vi "Fit Decay with Offset v2.vi"(0 "Y Array":dbl[](array[numeric]), 1 "X Array":dbl[](array[numeric]), 2 "Weights":dbl[](array[numeric]), 3 "Initial Parameters":dbl[](array[numeric]), 4 "Decay Fit Options":T2={"Show Fit Residuals"=TRUE, "Fit Model"=enum."1-Exponential", "Residual Type"=enum."Standard", "Max Decay Percentile"=0.0, "Min Decay Percentile"=0.0, "Show Full Decay"=TRUE, "Weights"=enum."Unweighted", "Fitting Method"=enum."Least Square", "Compute Parameter Uncertainties"=TRUE, "Periodic Boundaries"=TRUE, "Model Calculation"=enum."Simulation", "Period"=1.2500000000000001e-08, "Termination Criteria"={"Max Iterations"=0, "Max Function Calls"=0, "Max Time"=1000.0, "Function Tolerance"=1e-06, "Parameter Tolerance"=1e-06, "Gradient Tolerance"=0.0, "Min Lambda"=1e-06, "Max Lambda"=1e-06, "Initial Tick Count"=0}, "Offset Resolution"=1.2500000000000001e-08, "Use Local IRF"=TRUE, "Fitting Algorithm"=enum."Levenberg-Marquardt", "Show Confidence Interval "=TRUE, "Confidence Level"=95.0} {"Confidence Level" min=0.0 max=100.0; "Offset Resolution" min=0.0; "Period" min=0.0; "Min Decay Percentile" min=0.0 max=1.0; "Max Decay Percentile" min=0.0 max=100.0}, 5 "error in (no error)":errorcluster, 6 "f(x,a)":refnum<vi>, 7 "parameter bounds":T15, 8 "Data":variant, 9 "Decay Normalization Factor":dbl, 10 "Model Name":string, 11 "IRF Normalization Factor":dbl, 12 "Optimal Offset Selection Criterion":T1) -> (14 "Fit Output":T10={"best nonlinear fit"=[], "best fit parameters"=[], "R^2"=0.0, "RMSE"=0.0, "error out"={"status"=FALSE, "code"=0, "source"=""}, "Fitting Method"=enum."Least Square", "number of function calls"=0, "number of iterations"=0, "covariance"=[], "Chi 2"=0.0, "DOF"=0, "Fit Convergence Criterion"=enum."Continue", "Fitting Algorithm"=enum."Levenberg-Marquardt", "Weighted Fit"=enum."Unweighted", "Gradient"=0.0, "|Delta Chi 2|"=0.0, "|Delta Chi 2|/Chi 2"=0.0, "Max |Delta a| /|a|"=0.0, "Lambda"=-1.0, "RSS"=0.0, "AIC"=0.0, "BIC"=0.0, "Max number of function calls"=0, "Max number of iterations"=0, "IRF"={"X Array"=[], "Y Array"=[]}, "IRF Normalization Factor"=0.0, "Decay Normalization Factor"=0.0, "Number of offset fits"=0, "Weighted Chi2"=-1.0, "Unweighted Chi2"=-1.0}, 15 "Fit Aborted?":bool, 17 "Fit Results (Stats)":T9[](array[typedef]), 18 "C_00":dbl, 19 "error out":errorcluster)   [LabVIEW 2021, in "Fits.lvlib"]
uses:
  Fits.lvlib
  Non-linear Fit Output v4.ctl
  Nonlinear Fit Method.ctl
  <vilib>/Analysis/Matrix/Datatypes/RealMatrix.ctl
  Convergence Criteria.ctl
  Non-linear Fitting Algorithm.ctl
  Fit Weights Type v2.ctl
  Graphs/XY Graph/XY Graph Plot Data.ctl
  Fit Results (statistics).ctl
  Non-linear Fitting Method v2.ctl
  Decay Fit Options v4.ctl
  Decay Convolution/Decay Model.ctl
  Residual Type.ctl
  Fit Calculation Method.ctl
  Optimal Offset Selection Criterion.ctl
  Decay Fit Steps.ctl
  <vilib>/Analysis/Matrix/NI_Matrix.lvlib
  Graphs/XY Graph/XY Graph Add-Ons.lvlib
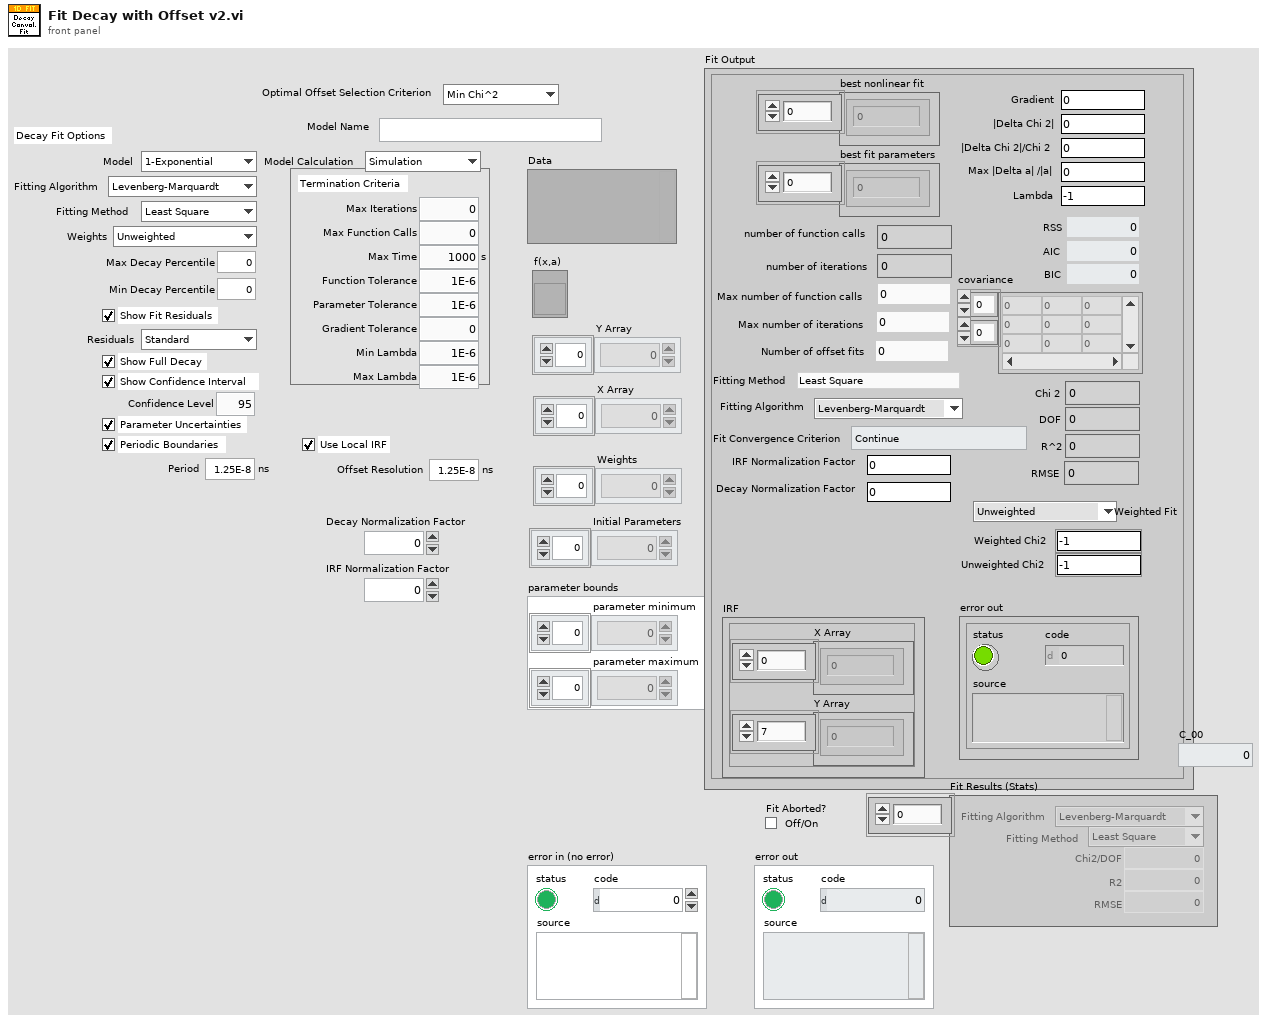
[diagram p1: front panel]
types:
  T1 = typedef "Fits.lvlib/Optimal Offset Selection Criterion.ctl" = enum16{"Min Chi^2", "Max R^2"}
  T2 = typedef "Fits.lvlib/Decay Fit Options v4.ctl" = cluster{"Show Fit Residuals":bool, "Fit Model":T3, "Residual Type":T4, "Max Decay Percentile":dbl, "Min Decay Percentile":dbl, "Show Full Decay":bool, "Weights":T5, "Fitting Method":T6, "Compute Parameter Uncertainties":bool, "Periodic Boundaries":bool, "Model Calculation":T7, "Period":dbl[unit], "Termination Criteria":cluster{"Max Iterations":i32, "Max Function Calls":i32, "Max Time":dbl[unit], "Function Tolerance":dbl, "Parameter Tolerance":dbl, "Gradient Tolerance":dbl, "Min Lambda":dbl, "Max Lambda":dbl, "Initial Tick Count":u32}, "Offset Resolution":dbl[unit], "Use Local IRF":bool, "Fitting Algorithm":T8, "Show Confidence Interval ":bool, "Confidence Level":dbl}
  T3 = typedef "Fits.lvlib/Decay Model.ctl" = enum16{"1-Exponential", "2-Exponentials"}
  T4 = typedef "Fits.lvlib/Residual Type.ctl" = enum16{"Standard", "Normalized", "Reduced"}
  T5 = typedef "Fits.lvlib/Fit Weights Type v2.ctl" = enum16{"Unweighted", "1/Variance (Neyman)", "1/Variance (Pearson)", "Best of All"}
  T6 = typedef "Fits.lvlib/Non-linear Fitting Method v2.ctl" = enum16{"Least Square", "Least Absolute Residual", "Bisquare", "MLE", "-", "Best of All"}
  T7 = typedef "Fits.lvlib/Fit Calculation Method.ctl" = enum16{"Simulation", "Convolution", "Integration"}
  T8 = typedef "Fits.lvlib/Non-linear Fitting Algorithm.ctl" = enum16{"Levenberg-Marquardt", "Trust-Region Dogleg"}
  T9 = typedef "Fits.lvlib/Fit Results (statistics).ctl" = cluster{"Chi2/DOF":dbl, "R2":dbl, "RMSE":dbl, "Fitting Method":T6, "Fitting Algorithm":T8}
  T10 = typedef "Fits.lvlib/Non-linear Fit Output v4.ctl" = cluster{"best nonlinear fit":dbl[], "best fit parameters":dbl[], "R^2":dbl, "RMSE":dbl, "error out":errorcluster, "Fitting Method":T11, "number of function calls":i32, "number of iterations":i32, "covariance":T12, "Chi 2":dbl, "DOF":i32, "Fit Convergence Criterion":T13, "Fitting Algorithm":T8, "Weighted Fit":T5, "Gradient":dbl, "|Delta Chi 2|":dbl, "|Delta Chi 2|/Chi 2":dbl, "Max |Delta a| /|a|":dbl, "Lambda":dbl, "RSS":dbl, "AIC":dbl, "BIC":dbl, "Max number of function calls":i32, "Max number of iterations":i32, "IRF":T14, "IRF Normalization Factor":dbl, "Decay Normalization Factor":dbl, "Number of offset fits":i32, "Weighted Chi2":dbl, "Unweighted Chi2":dbl}
  T11 = typedef "Fits.lvlib/Nonlinear Fit Method.ctl" = enum16{"Least Square", "Least Absolute Residual", "Bisquare", "MLE"}
  T12 = typedef "NI_Matrix.lvlib/RealMatrix.ctl" = dbl[][]
  T13 = typedef "Fits.lvlib/Convergence Criteria.ctl" = enum16{"Continue", "Tolerances Exceeded", "Max Time Exceeded", "Max Iterations Exceeded", "Max Function Evaluations Exceeded", "Scale Range Exceeded"}
  T14 = typedef "XY Graph Add-Ons.lvlib/XY Graph Plot Data.ctl" = cluster{"X Array":dbl[], "Y Array":dbl[]}
  T15 = cluster{"parameter minimum":dbl[], "parameter maximum":dbl[]}
  T16 = cluster{"Max Iterations":i32, "Max Function Calls":i32, "Max Time":dbl[unit], "Function Tolerance":dbl, "Parameter Tolerance":dbl, "Gradient Tolerance":dbl, "Min Lambda":dbl, "Max Lambda":dbl, "Initial Tick Count":u32}
  T17 = typedef "Fits.lvlib/Decay Fit Steps.ctl" = enum16{"Unweighted Fit", "Weighted Fit", "Best Fit"}
  T18 = cluster{"parameter minimum":dbl[], "parameter maximum":dbl[]}[]
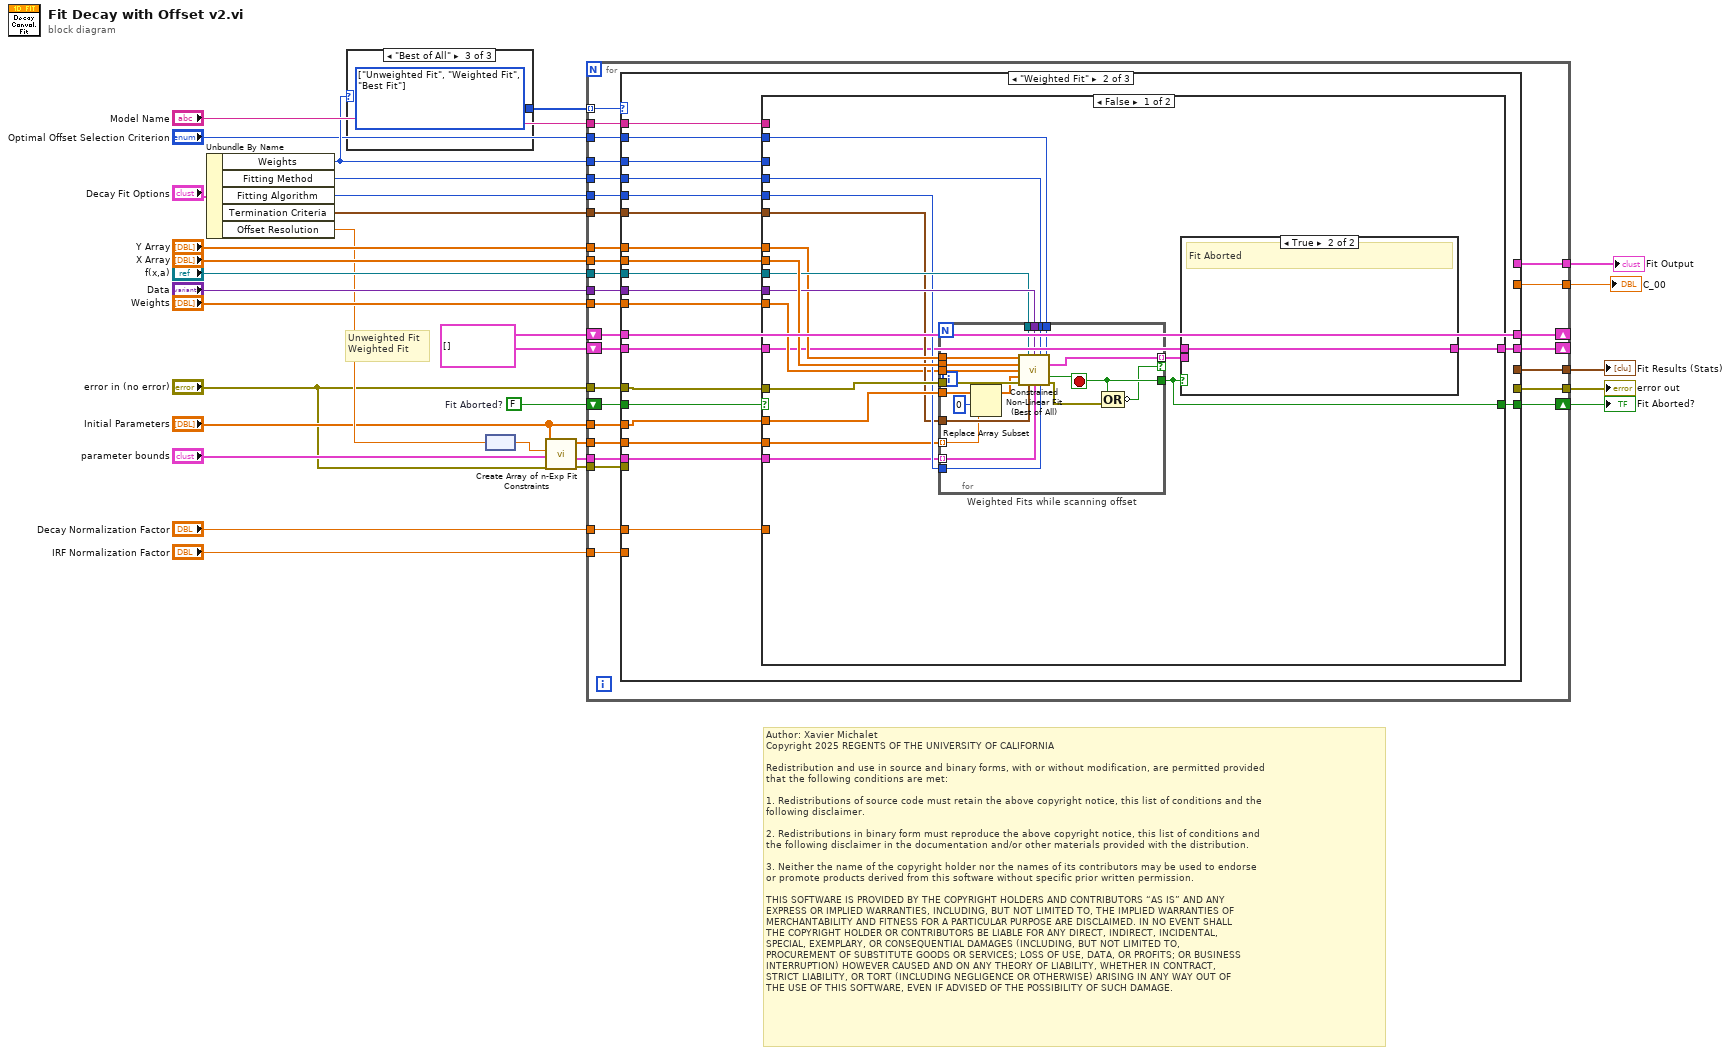
[diagram p0: block diagram]
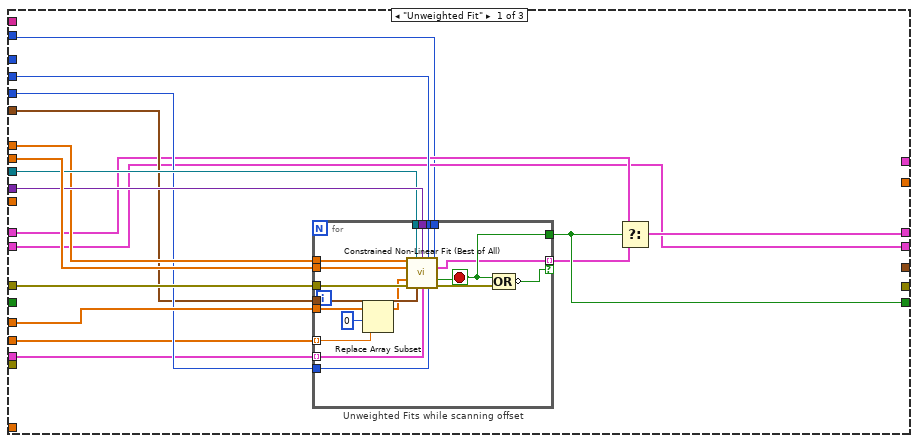
[diagram p2: hidden frame]
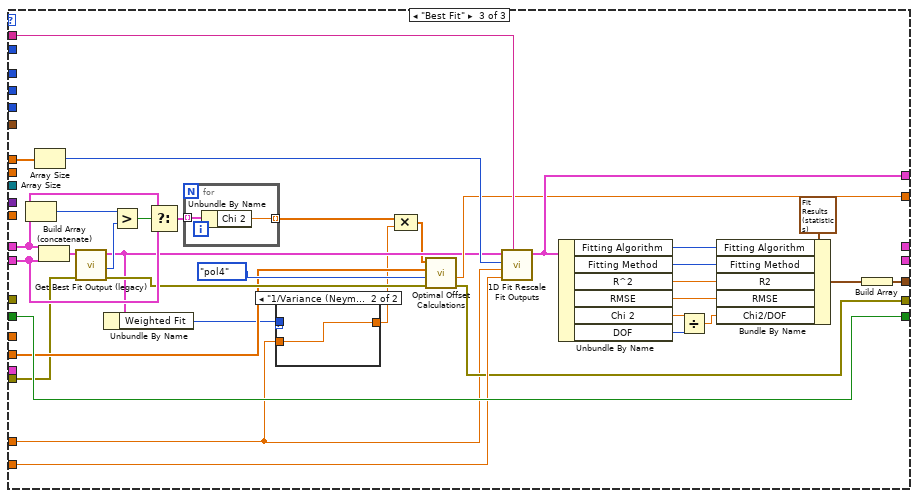
[diagram p5: hidden frame]
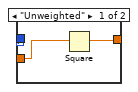
[diagram p6: hidden frame]
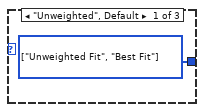
[diagram p7: hidden frame]
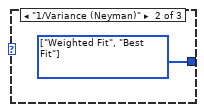
[diagram p8: hidden frame]
diagram:
  w14 = FALSE  # Fit Aborted?
  w11 = T10[] []
  # "Author: Xavier Michalet\nCopyright 2025 REGENTS OF THE UNIVERSITY OF CALIFORNIA\n\nRedistribution and use in source and binary forms, with or without modification, are permitted provided\nthat the following conditions are met:\n\n1. Redistributions of source code must retain the above copyright notice, this list of conditions and the\nfollowing disclaimer.\n\n2. Redistributions in binary form must reproduce the above copyright notice, this list of conditions and\nthe following disclaimer in the documentation and/or other materials provided with the distribution.\n\n3. Neither the name of the copyright holder nor the names of its contributors may be used to endorse \nor promote products derived from this software without specific prior written permission.\n\nTHIS SOFTWARE IS PROVIDED BY THE COPYRIGHT HOLDERS AND CONTRIBUTORS “AS IS” AND ANY \nEXPRESS OR IMPLIED WARRANTIES, INCLUDING, BUT NOT LIMITED TO, THE IMPLIED WARRANTIES OF\nMERCHANTABILITY AND FITNESS FOR A PARTICULAR PURPOSE ARE DISCLAIMED. IN NO EVENT SHALL\nTHE COPYRIGHT HOLDER OR CONTRIBUTORS BE LIABLE FOR ANY DIRECT, INDIRECT, INCIDENTAL, \nSPECIAL, EXEMPLARY, OR CONSEQUENTIAL DAMAGES (INCLUDING, BUT NOT LIMITED TO, \nPROCUREMENT OF SUBSTITUTE GOODS OR SERVICES; LOSS OF USE, DATA, OR PROFITS; OR BUSINESS\nINTERRUPTION) HOWEVER CAUSED AND ON ANY THEORY OF LIABILITY, WHETHER IN CONTRACT, \nSTRICT LIABILITY, OR TORT (INCLUDING NEGLIGENCE OR OTHERWISE) ARISING IN ANY WAY OUT OF\nTHE USE OF THIS SOFTWARE, EVEN IF ADVISED OF THE POSSIBILITY OF SUCH DAMAGE."
  # "Unweighted Fit\nWeighted Fit"
  n1 = Unbundle By Name("Decay Fit Options") -> ("Weights"=w16:T5, "Fitting Method"=w22:T6, "Fitting Algorithm"=w21:T8, "Termination Criteria"=w17:T16, "Offset Resolution"=w20:dbl[unit])
  n2 = case shown="\"Best of All\"" w16 {
    tunnel: [w31 w32 w33] -> w15
    frame "Unweighted", Default {
      w31 = T17[] [enum."Unweighted Fit", enum."Best Fit"] items=["Unweighted Fit", "Weighted Fit", "Best Fit"]
    }
    frame "1/Variance (Neyman)" {
      w32 = T17[] [enum."Weighted Fit", enum."Best Fit"] items=["Unweighted Fit", "Weighted Fit", "Best Fit"]
    }
    frame "Best of All" {
      w33 = T17[] [enum."Unweighted Fit", enum."Weighted Fit", enum."Best Fit"] items=["Unweighted Fit", "Weighted Fit", "Best Fit"]
    }
  }
  n3 = node(w20) -> (w9:dbl)
  n4 = call "Create Array of n-Exp Fit Constraints.vi"("Error In"="error in (no error)", "parameter bounds in"="parameter bounds", "Offset Resolution"=w9, "Guess Parameters in"="Initial Parameters") -> ("Error Out"=w1:errorcluster, "Array of parameter bounds"=w5:T18, "Guess Offset Array"=w7:dbl[])  [unwired: 5 in]
  n5 = for {
    tunnel: "Weights" -> [w62]
    tunnel: "X Array" -> [w61]
    tunnel: "Data" -> [w60]
    tunnel: "f(x,a)" -> [w59]
    tunnel: "Y Array" -> [w58]
    tunnel: [w57] -> w25
    tunnel: "error in (no error)" -> [w56]
    tunnel: [w55] -> w24
    tunnel: "Initial Parameters" -> [w54]
    tunnel: w16 -> [w53]
    tunnel: w22 -> [w52]
    tunnel: w21 -> [w51]
    tunnel: "Model Name" -> [w50]
    tunnel: "Decay Normalization Factor" -> [w49]
    tunnel: w17 -> [w48]
    tunnel: w15 -> [w47] mode=indexing
    shift-right: [w46] -> _
    shift-left: w11 -> [w45]
    shift-right: [w44] -> w13
    shift-left: w14 -> [w43]
    tunnel: "IRF Normalization Factor" -> [w42]
    shift-right: [w40] -> _
    shift-left: w11 -> [w41]
    tunnel: [w39] -> w10
    tunnel: w7 -> [w38]
    tunnel: w5 -> [w37]
    tunnel: [w36] -> w4
    tunnel: "Optimal Offset Selection Criterion" -> [w35]
    tunnel: w1 -> [w34]
    n6 = case shown="\"Weighted Fit\"" w47 {
      tunnel: w62 -> [_ w106 _]
      tunnel: w61 -> [w79 w118 _]
      tunnel: w60 -> [w78 w117 _]
      tunnel: w59 -> [w77 w116 _]
      tunnel: w58 -> [w76 w115 w180]
      tunnel: [_ _ w166] -> w57
      tunnel: [w67 w101 _] -> w40
      tunnel: w56 -> [w75 w114 _]
      tunnel: [_ _ w193] -> w55
      tunnel: w54 -> [w74 w113 _]
      tunnel: w53 -> [_ w112 _]
      tunnel: w52 -> [w73 w111 _]
      tunnel: w51 -> [w72 w110 _]
      tunnel: w50 -> [_ w109 w192]
      tunnel: w49 -> [_ w108 w161]
      tunnel: w48 -> [w71 w107 _]
      tunnel: [w66 w105 _] -> w46
      tunnel: w45 -> [w66 w104 w172]
      tunnel: [w70 w103 w191] -> w44
      tunnel: w43 -> [_ w102 w191]
      tunnel: w42 -> [_ _ w181]
      tunnel: w41 -> [w68 w101 w173]
      tunnel: [_ _ w177] -> w39
      tunnel: w38 -> [w64 w100 w169]
      tunnel: w37 -> [w65 w99 _]
      tunnel: [_ _ w167] -> w36
      tunnel: w35 -> [w63 w98 _]
      tunnel: w34 -> [_ _ w160]
      frame "Unweighted Fit" {
        n7 = for "Unweighted Fits while scanning offset" {
          tunnel: w77 -> [w97]
          tunnel: [w81] -> w69 mode=indexing if=w84
          tunnel: w76 -> [w95]
          tunnel: w79 -> [w94]
          tunnel: w65 -> [w85] mode=indexing
          tunnel: w73 -> [w93]
          tunnel: w74 -> [w92]
          tunnel: w78 -> [w91]
          tunnel: w71 -> [w90]
          tunnel: w75 -> [w96]
          tunnel: [w89] -> w70
          tunnel: w72 -> [w86]
          tunnel: w64 -> [w82] mode=indexing
          tunnel: w63 -> [w80]
          stop <- w89 stop-if-true
          n8 = Replace Array Subset(array=w92, new element=w82, index=0) -> (w88:dbl[])
          n9 = call "Constrained Non-Linear Fit (Best of All).vi"("Y Array"=w95, "f(x,a)"=w97, "Data"=w91, "Fitting Method"=w93, "Optimal Offset Selection Criterion"=w80, "X Array"=w94, "Guess Fitted Parameters"=w88, "error in (no error)"=w96, "Termination Criteria"=w90, "Fitted parameter bounds"=w85, "Fitting Algorithm"=w86) -> ("Fit Output"=w81:T10, "Fit Aborted?"=w89:bool, "Error Out"=w83:errorcluster)  [unwired: 1 in, 1 out]
          n10 = Compound Arithmetic op=OR(w89, w83) -> (invert w84:bool)
        }
        n11 = Select(t=w68, s=w70, f=w69) -> (s? t:f=w67:T10[])
      }
      frame "Weighted Fit" {
        n12 = case shown="False" w102 {
          selector: w102 -> [_ w157]
          tunnel: w118 -> [w135 _]
          tunnel: w117 -> [w134 _]
          tunnel: w116 -> [w133 _]
          tunnel: w115 -> [w132 _]
          tunnel: w114 -> [w130 _]
          tunnel: w113 -> [w129 _]
          tunnel: w112 -> [_ _]
          tunnel: w111 -> [w128 _]
          tunnel: w110 -> [w127 _]
          tunnel: w109 -> [_ _]
          tunnel: w108 -> [_ _]
          tunnel: w107 -> [w126 _]
          tunnel: w106 -> [w125 _]
          tunnel: [w124 w158] -> w105
          tunnel: w104 -> [w122 w158]
          tunnel: [w123 w157] -> w103
          tunnel: w100 -> [w121 _]
          tunnel: w99 -> [w120 _]
          tunnel: w98 -> [w119 _]
          frame False {
            n13 = for "Weighted Fits while scanning offset" {
              tunnel: w133 -> [w156]
              tunnel: [w139] -> w131 mode=indexing if=w142
              tunnel: w132 -> [w154]
              tunnel: w135 -> [w153]
              tunnel: w120 -> [w143] mode=indexing
              tunnel: w128 -> [w152]
              tunnel: w129 -> [w151]
              tunnel: w134 -> [w150]
              tunnel: w126 -> [w149]
              tunnel: w130 -> [w155]
              tunnel: [w148] -> w123
              tunnel: w121 -> [w146] mode=indexing
              tunnel: w127 -> [w144]
              tunnel: w125 -> [w140]
              tunnel: w119 -> [w138]
              stop <- w148 stop-if-true
              n14 = Replace Array Subset(array=w151, new element=w146, index=0) -> (w147:dbl[])
              n15 = call "Constrained Non-Linear Fit (Best of All).vi"("Y Array"=w154, "f(x,a)"=w156, "Data"=w150, "Fitting Method"=w152, "Optimal Offset Selection Criterion"=w138, "X Array"=w153, "Weights"=w140, "Guess Fitted Parameters"=w147, "error in (no error)"=w155, "Termination Criteria"=w149, "Fitted parameter bounds"=w143, "Fitting Algorithm"=w144) -> ("Fit Output"=w139:T10, "Fit Aborted?"=w148:bool, "Error Out"=w141:errorcluster)  [unwired: 1 out]
              n16 = Compound Arithmetic op=OR(w148, w141) -> (invert w142:bool)
            }
            n17 = case shown="True" w123 {
              tunnel: w131 -> [w136 _]
              tunnel: [w136 w137] -> w124
              tunnel: w122 -> [_ w137]
              frame False {
                # "Fit not aborted during weighted fit"
              }
              frame True {
                # "Fit Aborted"
              }
            }
          }
          frame True {
          }
        }
      }
      frame "Best Fit" {
        n18 = Array Size(array=w173) -> (size(s)=w176:i32)
        n19 = Array Size(array=w180) -> (size(s)=w179:i32)
        n20 = Build Array (concatenate)(w173, w172) -> (w178:T10[])
        n21 = call "Get Best Fit Output (legacy).vi"("error in"=w160, "Array of Fit Outputs"=w178) -> ("Error Out"=w171:errorcluster, "min index"=w175:i32, "Best Fit Output"=w165:T10)  [unwired: 7 in]
        n22 = Unbundle By Name(w165) -> ("Weighted Fit"=w159:T5)
        n23 = Greater?(x=w176, y=w175) -> (0:w174:bool)
        n24 = Select(t=w173, s=w174, f=w172) -> (s? t:f=w168:T10[])
        n25 = for {
          tunnel: w168 -> [w198] mode=indexing
          tunnel: [w197] -> w163 mode=indexing
          n26 = Unbundle By Name(w198) -> ("Chi 2"=w197:dbl)
        }
        n27 = case shown="\"1/Variance (Neyman)\", Default" w159 {
          tunnel: [w194 w196] -> w164
          tunnel: w159 -> [_ _]
          tunnel: w161 -> [w195 w196]
          frame "Unweighted" {
            n28 = Square(x=w195) -> (x^2=w194:dbl)
          }
          frame "1/Variance (Neyman)", Default {
          }
        }
        n29 = Compound Arithmetic op=MULTIPLY(w163, w164) -> (w162:dbl[])
        n30 = call "Optimal Offset Calculations.vi"("Error In"=w171, "Polynomial"=enum16{"pol2", "pol4"}."pol4", "Offset Array"=w169, "Chi^2 Array"=w162) -> ("Error Out"=w166:errorcluster, "C00"=w167:dbl)  [unwired: 2 in, 4 out]
        n31 = call "1D Fit Rescale Fit Outputs.vi"("Model Name"=w192, "IRF Normalization Factor"=w181, "Decay Normalization Factor"=w161, "# Points"=w179, "Fit Output in"=w165) -> ("Fit Output out"=w177:T10)  [unwired: 6 in]
        n32 = Unbundle By Name(w177) -> ("Fitting Algorithm"=w184:T8, "Fitting Method"=w188:T11, "R^2"=w187:dbl, "RMSE"=w186:dbl, "Chi 2"=w185:dbl, "DOF"=w183:i32)
        n33 = Divide(x=w185, y=w183) -> (x/y=w182:dbl)
        n34 = Bundle By Name(cluster=T9 {"Chi2/DOF"=0.0, "R2"=0.0, "RMSE"=0.0, "Fitting Method"=enum."Least Square", "Fitting Algorithm"=enum."Levenberg-Marquardt"} ("Fit Results (Stats)"), "Fitting Algorithm"=w184, "Fitting Method"=w188, "R2"=w187, "RMSE"=w186, "Chi2/DOF"=w182) -> (w189:T9)
        n35 = Build Array(w189) -> (w193:T9[])
      }
    }
  }
  "error out" <- w25
  "Fit Output" <- w10
  "Fit Aborted?" <- w13
  "Fit Results (Stats)" <- w24
  "C_00" <- w4
